vi "waveform2X.vi"(6 "error in":errorcluster, 9 "use t0":bool, 10 "waveform":waveform(dbl)) -> (2 "X":dbl[](array[numeric]), 4 "error out":errorcluster, 5 "end":dbl, 7 "start":dbl)   [LabVIEW 2015]
uses:
  <vilib>/Utility/error.llb/DialogType.ctl
  <vilib>/Analysis/1siggen.llb/Ramp Pattern by Samples.vi
  <vilib>/Analysis/NI_AALBase.lvlib
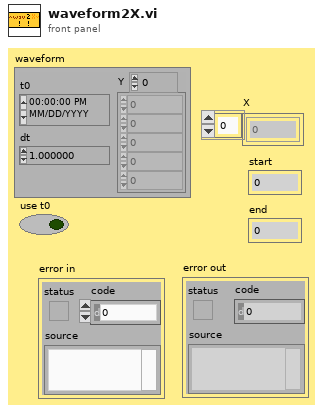
[diagram p1: front panel]
types:
  T1 = typedef "DialogType.ctl" = u16
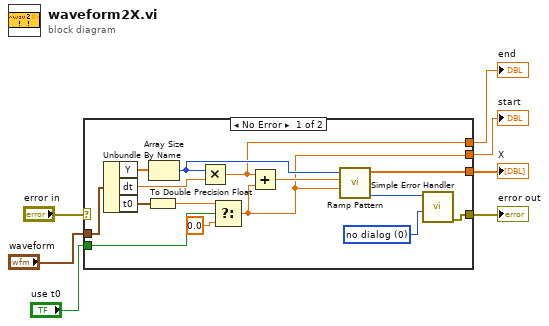
[diagram p0: block diagram]
diagram:
  n1 = case shown="No Error" "error in" {
    selector: "error in" -> [_ w23]
    tunnel: "waveform" -> [w18 _]
    tunnel: [w15 w23] -> w6
    tunnel: [w14 _] -> w5
    tunnel: [w10 _] -> w3
    tunnel: [w13 _] -> w2
    tunnel: "use t0" -> [w8 _]
    frame No Error {
      w16 = T1 0 items=["no dialog", "OK message", "continue or stop message", "OK message + warnings", "continue/stop + warnings"] ("type of dialog (OK msg:1)")
      n2 = Unbundle By Name(w18) -> ("Y"=w20:dbl[], "dt"=w21:dbl, "t0"=w19:timestamp)
      n3 = To Double Precision Float(number=w19) -> (double precision float=w11:dbl)
      n4 = Array Size(array=w20) -> (size(s)=w22:i32)
      n5 = Multiply(x=w22, y=w21) -> (x*y=w13:dbl)
      n6 = Select(t=w11, s=w8, f=0.0) -> (s? t:f=w10:dbl)
      n7 = Add(x=w13, y=w10) -> (x+y=w12:dbl)
      n8 = call-poly <vilib>:"Ramp Pattern.vi"("start"=w10, "end"=w12, "samples"=w22) -> ("error"=w17:i32, "Ramp Pattern"=w14:dbl[])  [unwired: 7 in]
      n9 = call <vilib>:"Simple Error Handler.vi"("error code (no error:0)"=w17, "type of dialog (OK msg:1)"=w16) -> ("error out"=w15:errorcluster)  [unwired: 3 in, 4 out]
    }
    frame Error {
    }
  }
  "error out" <- w6
  "X" <- w5
  "end" <- w2
  "start" <- w3
